vi "Empty_tree.vi"(8 "error in (no error)":errorcluster, 11 "Script_Tree":refnum<vi>) -> (0 "error out":errorcluster, 3 "Script_Tree":refnum<vi>)   [LabVIEW 2024, in "Setting_Screen.lvlib"]
uses:
  Setting_Screen.lvlib
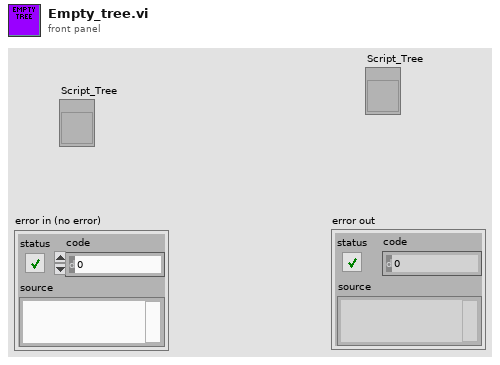
[diagram p1: front panel]
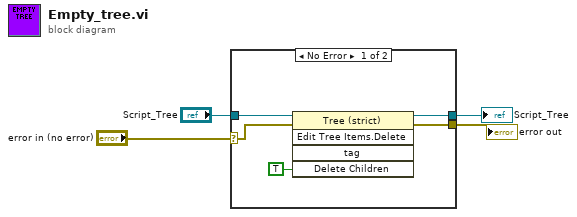
[diagram p0: block diagram]
diagram:
  n1 = case shown="No Error" "error in (no error)" {
    selector: "error in (no error)" -> [w8 w11]
    tunnel: "Script_Tree" -> [w9 w10]
    tunnel: [w7 w10] -> w2
    tunnel: [w6 w11] -> w1
    frame No Error {
      n2 = invoke class="Tree (strict)" method="Edit Tree Items.Delete"(reference=w9, error in=w8, "Delete Children"=TRUE ("Delete Children?")) -> (reference out=w7:refnum<vi>, error out=w6:errorcluster)  [unwired: 2 in, 3 out]
    }
    frame Error {
    }
  }
  "Script_Tree" <- w2
  "error out" <- w1
